vi "Scale GUI.vi"(0 "Clust Refnum":refnum<vi>) -> ()   [LabVIEW 2015]
uses:
  conversion.ctl
  DAQ configuration/scale type.ctl
  correspondence table.ctl
  pH/pH scale.ctl
  Dissolved Oxygen/DO scale.ctl
  Spectrophotometer/Photometer calibration data.ctl
panel:
  out "size(s)":i32
  # "C"
  # "kPa"
  # "C"
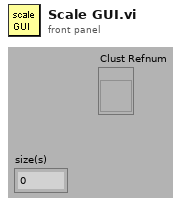
[diagram p1: front panel]
types:
  T1 = typedef "conversion.ctl" = cluster{"conversion matrix":sgl[][], "units":string, "name":string, "scale type":T2, "offset (volts)":dbl, "second channel":i8, "correspondence table":T3, "offset (physical units)":dbl, "pH scale":T4, "D.O.":T5, "Photometer data":T6}
  T2 = typedef "scale type.ctl" = enum16{"Volts", "Polynomial", "Correspondence Table", "pH", "Dissolved Oxygen", "Quadratic", "Photometer"}
  T3 = typedef "correspondence table.ctl" = cluster{"physical units":dbl, "volts":dbl}[]
  T4 = typedef "pH scale.ctl" = cluster{"Buffers":cluster{"Buffer":dbl, "Calibrated":bool, "V/T":dbl}[], "Temperature":dbl}
  T5 = typedef "DO scale.ctl" = cluster{"Temperature":dbl, "K":dbl, "barometric pressure":dbl}
  T6 = typedef "Photometer calibration data.ctl" = cluster{"Dark Voltage":dbl, "Blank Voltage":dbl, "Standards":cluster{"Concentration":dbl, "Voltage":dbl}[]}
  T7 = cluster{"Controls[][0]":refnum<vi>, "Controls[][1]":refnum<vi>, "Controls[][2]":refnum<vi>, "Controls[][3]":refnum<vi>, "Controls[][4]":refnum<vi>, "Controls[][5]":refnum<vi>, "Controls[][6]":refnum<vi>, "Controls[][7]":refnum<vi>, "Controls[][8]":refnum<vi>, "Controls[][9]":refnum<vi>, "Controls[][10]":refnum<vi>}
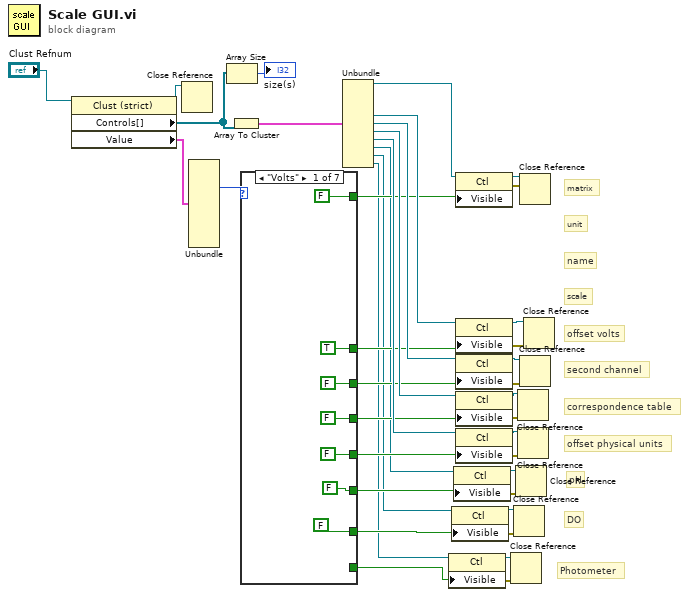
[diagram p0: block diagram]
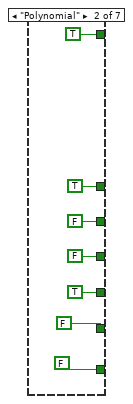
[diagram p2: hidden frame]
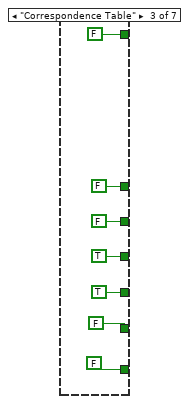
[diagram p3: hidden frame]
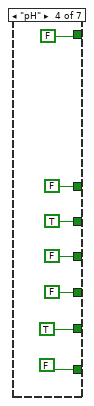
[diagram p4: hidden frame]
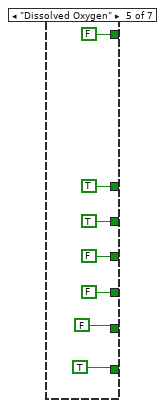
[diagram p5: hidden frame]
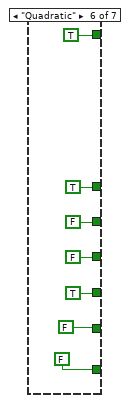
[diagram p6: hidden frame]
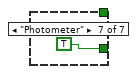
[diagram p7: hidden frame]
diagram:
  # "Photometer"
  # "DO"
  # "pH"
  # "offset physical units"
  # "correspondence table"
  # "second channel"
  # "offset volts"
  # "scale"
  # "name"
  # "unit"
  # "matrix"
  n1 = property class="Clust (strict)"(reference="Clust Refnum") -> (reference out=w24:refnum<vi>, "Controls[]"=w37:refnum<vi>[], "Value"=w39:T1)  [unwired: 1 in, 1 out]
  n2 = Close Reference(reference=w24) -> ()  [unwired: 1 in, 1 out]
  n3 = Unbundle(w39) -> ("scale type"=w38:T2)  [unwired: 10 out]
  n4 = Array Size(array=w37) -> (size(s)=→"size(s)":i32)
  n5 = Array To Cluster(array=w37) -> (cluster=w35:T7)
  n6 = case shown="\"Volts\"" w38 {
    tunnel: [TRUE TRUE FALSE FALSE TRUE TRUE _] -> w29
    tunnel: [FALSE FALSE FALSE TRUE TRUE FALSE _] -> w28
    tunnel: [FALSE FALSE TRUE FALSE FALSE FALSE _] -> w27
    tunnel: [FALSE TRUE TRUE FALSE FALSE TRUE _] -> w26
    tunnel: [FALSE TRUE FALSE FALSE FALSE TRUE _] -> w25
    tunnel: [FALSE FALSE FALSE TRUE FALSE FALSE _] -> w11
    tunnel: [FALSE FALSE FALSE FALSE TRUE FALSE _] -> w7
    tunnel: [_ _ _ _ _ _ TRUE] -> w2
    frame "Volts" {
    }
    frame "Polynomial" {
    }
    frame "Correspondence Table" {
    }
    frame "pH" {
    }
    frame "Dissolved Oxygen" {
    }
    frame "Quadratic" {
    }
    frame "Photometer" {
    }
  }
  n7 = Unbundle(w35) -> ("Controls[][0]"=w34:refnum<vi>, "Controls[][4]"=w33:refnum<vi>, "Controls[][5]"=w32:refnum<vi>, "Controls[][6]"=w31:refnum<vi>, "Controls[][7]"=w30:refnum<vi>, "Controls[][8]"=w12:refnum<vi>, "Controls[][9]"=w8:refnum<vi>, "Controls[][10]"=w3:refnum<vi>)  [unwired: 3 out]
  n8 = property class="Ctl"(reference=w3, "Visible"=w2) -> (reference out=w1:refnum<vi>, error out=w4:errorcluster)  [unwired: 1 in]
  n9 = property class="Ctl"(reference=w8, "Visible"=w7) -> (reference out=w6:refnum<vi>, error out=w9:errorcluster)  [unwired: 1 in]
  n10 = property class="Ctl"(reference=w12, "Visible"=w11) -> (reference out=w10:refnum<vi>, error out=w13:errorcluster)  [unwired: 1 in]
  n11 = property class="Ctl"(reference=w34, "Visible"=w25) -> (reference out=w15:refnum<vi>, error out=w14:errorcluster)  [unwired: 1 in]
  n12 = property class="Ctl"(reference=w33, "Visible"=w29) -> (reference out=w22:refnum<vi>, error out=w23:errorcluster)  [unwired: 1 in]
  n13 = property class="Ctl"(reference=w32, "Visible"=w28) -> (reference out=w20:refnum<vi>, error out=w21:errorcluster)  [unwired: 1 in]
  n14 = property class="Ctl"(reference=w31, "Visible"=w27) -> (reference out=w18:refnum<vi>, error out=w19:errorcluster)  [unwired: 1 in]
  n15 = property class="Ctl"(reference=w30, "Visible"=w26) -> (reference out=w16:refnum<vi>, error out=w17:errorcluster)  [unwired: 1 in]
  n16 = Close Reference(reference=w1, error in (no error)=w4) -> ()  [unwired: 1 out]
  n17 = Close Reference(reference=w6, error in (no error)=w9) -> ()  [unwired: 1 out]
  n18 = Close Reference(reference=w10, error in (no error)=w13) -> ()  [unwired: 1 out]
  n19 = Close Reference(reference=w18, error in (no error)=w19) -> ()  [unwired: 1 out]
  n20 = Close Reference(reference=w16, error in (no error)=w17) -> ()  [unwired: 1 out]
  n21 = Close Reference(reference=w15, error in (no error)=w14) -> ()  [unwired: 1 out]
  n22 = Close Reference(reference=w20, error in (no error)=w21) -> ()  [unwired: 1 out]
  n23 = Close Reference(reference=w22, error in (no error)=w23) -> ()  [unwired: 1 out]
